vi "Commit Build Settings.vi"(8 "error in (no error)":errorcluster, 11 "DLL in":refnum<class "NI_AB_API_DLL.lvclass">) -> (0 "error out":errorcluster, 3 "DLL out":refnum<class "NI_AB_API_DLL.lvclass">)   [LabVIEW 2020, in "NI_AB_API_DLL.lvclass"]
uses:
  <vilib>/AppBuilder/AB_API/DLL/NI_AB_API_DLL.lvclass
  <vilib>/AppBuilder/AB_API/DLL/NI_AB_API_DLL.lvclass/NI_AB_API_DLL.ctl
  <vilib>/AppBuilder/AB_API/Application/NI_AB_API_Application.lvclass
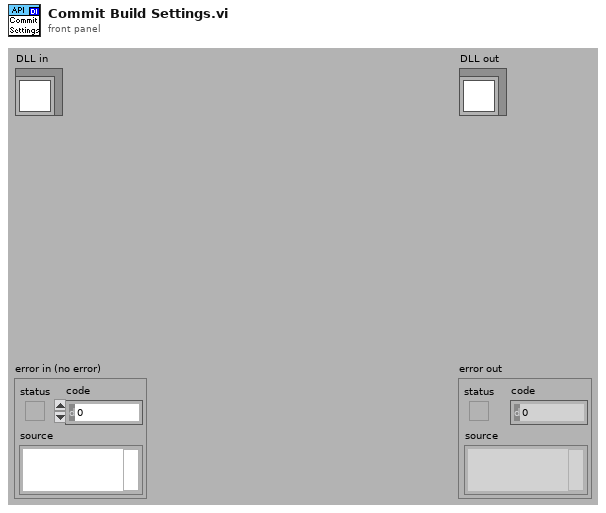
[diagram p1: front panel]
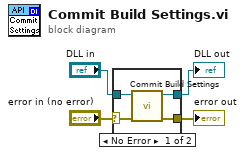
[diagram p0: block diagram]
diagram:
  n1 = case shown="No Error" "error in (no error)" {
    selector: "error in (no error)" -> [w6 w10]
    tunnel: [w5 w10] -> w3
    tunnel: [w7 w9] -> w1
    tunnel: "DLL in" -> [w8 w9]
    frame No Error {
      n2 = call-parent "Commit Build Settings.vi"("error in (no error)"=w6, "Build in"=w8) -> ("error out"=w5:errorcluster, "Build out"=w7:refnum<class "NI_AB_API_DLL.lvclass">)  [unwired: 8 in]
    }
    frame Error {
    }
  }
  "error out" <- w3
  "DLL out" <- w1
